vi "Initialize Logging Data.vi"(8 "error in (no error)":errorcluster, 11 "Device Reference in":T2 format="%.0x") -> (0 "error out":errorcluster, 2 "Logging Data":T1 {"Error Code Data Refnum" format="%.0x"; "System Channel Refnums" format="%.0x"; "Block Data Refnums"."Data Reference" format="%.0x"}, 3 "Device Reference out":T2=18446744073709551615 format="%.0x")   [LabVIEW 2019, in "Telemetry Engine.lvlib"]
uses:
  Telemetry Engine.lvlib
  <vilib>/NI VeriStand/Custom Device API/Custom Device Item Ref.ctl
  Types/Engine Logging Data.ctl
  <vilib>/NI VeriStand/Custom Device API/Block Data Reference.ctl
  <vilib>/NI VeriStand/Custom Device API/Data Reference.ctl
  <vilib>/NI VeriStand/Custom Device API/Data Access Type.ctl
  Shared/Constants.vi
  <vilib>/NI VeriStand/Custom Device Tools/Custom Device Utility Library/NI VeriStand - Search for Item by GUID.vi
  <vilib>/NI VeriStand/Custom Device Tools/Custom Device Utility Library/NI VeriStand - Search for Item by Property.vi
  <vilib>/NI VeriStand/Custom Device API/Get Item Property (String Array).vi
  <vilib>/NI VeriStand/Custom Device API/Custom Device API.lvlib
  <vilib>/NI VeriStand/Custom Device Tools/Custom Device Utility Library/Custom Device Utility Library.lvlib
  Shared/Telemetry Shared.lvlib
  <vilib>/NI VeriStand/Custom Device API/Get Item Property (Boolean).vi
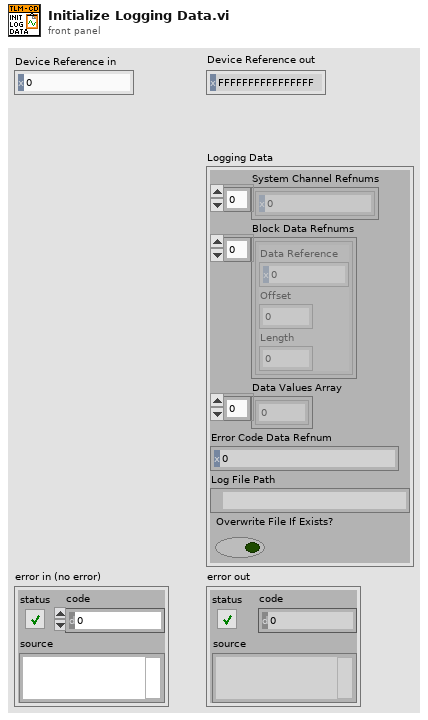
[diagram p1: front panel]
types:
  T1 = typedef "Telemetry Engine.lvlib/Engine Logging Data.ctl" = cluster{"System Channel Refnums":T2[], "Block Data Refnums":T3[], "Data Values Array":dbl[], "Error Code Data Refnum":T4, "Log File Path":path, "Overwrite File If Exists?":bool}
  T2 = typedef "Custom Device API.lvlib/Custom Device Item Ref.ctl" = u64
  T3 = typedef "Custom Device API.lvlib/Block Data Reference.ctl" = cluster{"Data Reference":T4, "Offset":u64, "Length":u64}
  T4 = typedef "Custom Device API.lvlib/Data Reference.ctl" = i32
  T5 = typedef "Custom Device API.lvlib/Data Access Type.ctl" = enum16{"Read", "Write"}
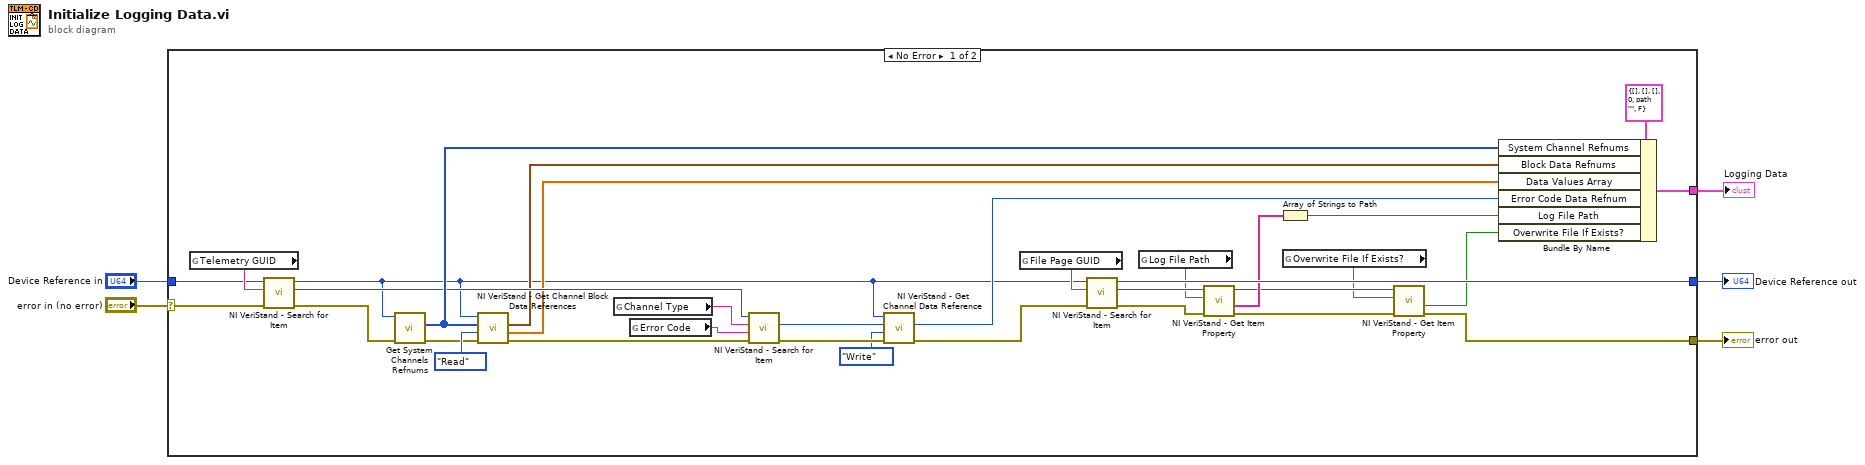
[diagram p0: block diagram]
diagram:
  n1 = case shown="No Error" "error in (no error)" {
    selector: "error in (no error)" -> [w29 w40]
    tunnel: "Device Reference in" -> [w30 w39]
    tunnel: [w23 w39] -> w4
    tunnel: [w6 w40] -> w3
    tunnel: [w36 _] -> w1
    frame No Error {
      n2 = global read "Constants.vi" "Telemetry GUID"() -> (w31:string)
      n3 = call-poly <vilib>:"NI VeriStand - Search for Item.vi"("error in"=w29, "Item GUID"=w31, "Section Ref in"=w30) -> ("error out"=w26:errorcluster, "Item Ref"=w25:T2, "Section Ref out"=w13:T2)  [unwired: 5 in, 1 out]
      n4 = call "Get System Channels Refnums.vi"("error in (no error)"=w26, "Item Ref in"=w13) -> ("error out"=w28:errorcluster, "System Channel Refs"=w37:T2[])  [unwired: 7 in, 1 out]
      n5 = call <vilib>:"NI VeriStand - Get Channel Block Data References.vi"("error in (no error)"=w28, "Access"=Data_Access_Type."Read", "Channel Refs"=w37, "Device Ref in"=w13) -> ("error out"=w27:errorcluster, "Values Array"=w15:dbl[], "Block Data Refs"=w14:T3[])  [unwired: 4 in, 1 out]
      n6 = global read "Constants.vi" "Channel Type"() -> (w12:string)
      n7 = global read "Constants.vi" "Error Code"() -> (w11:string)
      n8 = call-poly <vilib>:"NI VeriStand - Search for Item.vi"("error in"=w27, "Property Value"=w11, "Property Name"=w12, "Section Ref in"=w25) -> ("error out"=w34:errorcluster, "Item Ref"=w33:T2)  [unwired: 4 in, 2 out]
      n9 = call <vilib>:"NI VeriStand - Get Channel Data Reference.vi"("error in (no error)"=w34, "Access"=Data_Access_Type."Write", "Channel Ref in"=w33, "Device Ref in"=w13) -> ("error out"=w22:errorcluster, "Channel Data Reference"=w24:T4)  [unwired: 5 in, 1 out]
      n10 = global read "Constants.vi" "File Page GUID"() -> (w21:string)
      n11 = call-poly <vilib>:"NI VeriStand - Search for Item.vi"("error in"=w22, "Item GUID"=w21, "Section Ref in"=w13) -> ("error out"=w18:errorcluster, "Item Ref"=w20:T2, "Section Ref out"=w23:T2)  [unwired: 5 in, 1 out]
      n12 = global read "Constants.vi" "Log File Path"() -> (w19:string)
      n13 = call-poly <vilib>:"NI VeriStand - Get Item Property.vi"("error in (no error)"=w18, "Property Name"=w19, "Item Ref in"=w20) -> ("error out"=w9:errorcluster, "Value"=w17:string[], "Item Ref out"=w10:T2)  [unwired: 5 in, 1 out]
      n14 = Array of Strings to Path(0:w17) -> (2:w16:path)  [unwired: 1 in]
      n15 = global read "Constants.vi" "Overwrite File If Exists?"() -> (w8:string)
      n16 = call-poly <vilib>:"NI VeriStand - Get Item Property.vi"("error in (no error)"=w9, "Property Name"=w8, "Item Ref in"=w10) -> ("error out"=w6:errorcluster, "Value"=w7:bool)  [unwired: 5 in, 2 out]
      n17 = Bundle By Name(cluster=T1 {"System Channel Refnums"=[], "Block Data Refnums"=[], "Data Values Array"=[], "Error Code Data Refnum"=0, "Log File Path"=path "", "Overwrite File If Exists?"=FALSE} ("Logging Data"), "System Channel Refnums"=w37, "Block Data Refnums"=w14, "Data Values Array"=w15, "Error Code Data Refnum"=w24, "Log File Path"=w16, "Overwrite File If Exists?"=w7) -> (w36:T1)
    }
    frame Error {
    }
  }
  "error out" <- w3
  "Device Reference out" <- w4
  "Logging Data" <- w1
